vi "FGV_DataPackerTimingMetrics.vi"(7 "?":T1, 9 "% Time Packing (Serializing Queued Data)":dbl(knob) scale=0.0..100.0, 10 "Time Bundling Data (Reading from Queue into LV structures)":dbl(knob) scale=0.0..100.0, 11 "Time since last sleep (ms)":dbl(knob) scale=1.0..1000.0) -> (1 "% Time Packing (Serializing Queued Data)":dbl(knob) scale=0.0..100.0, 2 "Time Bundling Data (Reading from Queue into LV structures)":dbl(knob) scale=0.0..100.0, 3 "Time since last sleep (ms)":dbl(knob) scale=1.0..1000.0)   [LabVIEW 2018, in "feGEM DataPacker.lvlib"]
uses:
  feGEM DataPacker.lvlib
  Set_And_Get_Enum.ctl
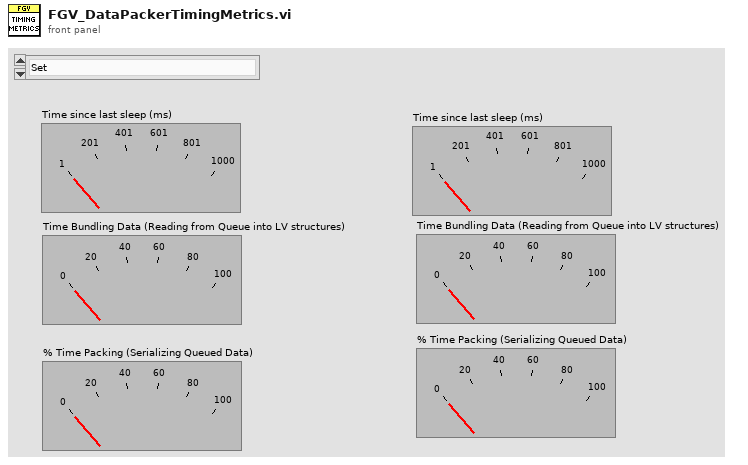
[diagram p1: front panel]
types:
  T1 = typedef "feGEM DataPacker.lvlib/Set_And_Get_Enum.ctl" = enum16{"Set", "Get"}
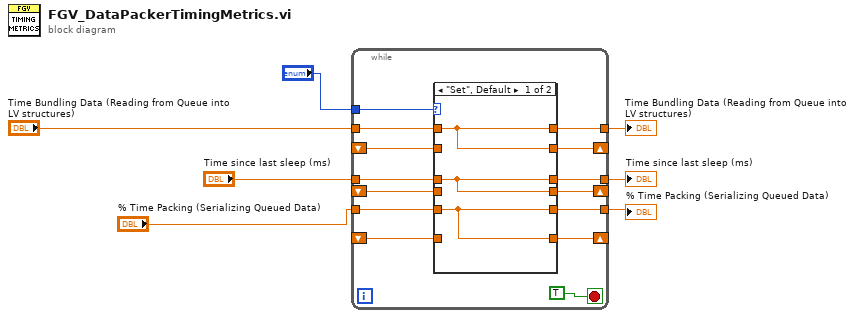
[diagram p0: block diagram]
diagram:
  n1 = while {
    tunnel: [w20] -> w2
    tunnel: "Time since last sleep (ms)" -> [w19]
    tunnel: "Time Bundling Data (Reading from Queue into LV structures)" -> [w16]
    tunnel: "% Time Packing (Serializing Queued Data)" -> [w18]
    tunnel: [w9] -> w4
    tunnel: [w17] -> w3
    shift-right: [w15] -> _
    shift-left: _ -> [w10]
    shift-right: [w14] -> _
    shift-left: _ -> [w11]
    shift-right: [w13] -> _
    shift-left: _ -> [w12]
    tunnel: "?" -> [w8]
    stop <- TRUE stop-if-true
    n2 = case shown="\"Set\", Default" w8 {
      tunnel: [w24 w27] -> w20
      tunnel: w19 -> [w24 _]
      tunnel: w18 -> [w22 _]
      tunnel: [w23 w26] -> w17
      tunnel: w16 -> [w23 _]
      tunnel: [w23 w26] -> w15
      tunnel: [w24 w27] -> w14
      tunnel: [w22 w25] -> w13
      tunnel: w12 -> [_ w25]
      tunnel: w11 -> [_ w27]
      tunnel: w10 -> [_ w26]
      tunnel: [w22 w25] -> w9
      frame "Set", Default {
      }
      frame "Get" {
      }
    }
  }
  "% Time Packing (Serializing Queued Data)" <- w4
  "Time Bundling Data (Reading from Queue into LV structures)" <- w3
  "Time since last sleep (ms)" <- w2
